vi "Do on Error.vi"(8 "error in (no error)":errorcluster, 11 "Debug UI in":refnum<class "Debug UI.lvclass">) -> ()   [LabVIEW 2018, in "Assert API Components.lvlib" / "Log Assert Core.lvlib" / "Debug UI.lvclass"]
doc: "Dynamic dispatch vi to be overriden by file or debug UI - takes the action to pass the error and handle it as required."
uses:
  Debug UI.lvclass
  C:/Program Files (x86)/National Instruments/LabVIEW 2018/vi.lib/ActorFramework/Actor/Actor.lvclass
  <vilib>/ActorFramework/Message Enqueuer/Message Enqueuer.lvclass
  Debug UI Messages/Error Data Msg/Error Data Msg.lvclass/Error Data Msg.ctl
  <vilib>/ActorFramework/Message Enqueuer/Message Enqueuer.lvclass/Message Enqueuer.ctl
  <vilib>/ActorFramework/Message Enqueuer/Enqueue.vi
  Debug UI Messages/Error Data Msg/Error Data Msg.lvclass
  C:/Program Files (x86)/National Instruments/LabVIEW 2018/vi.lib/ActorFramework/Message/Message.lvclass
  <vilib>/Utility/LVClass/Get LV Class Name.vi
  <resource>/AFDebug/Generate Trace for Message.vi
  <vilib>/ActorFramework/Message Priority Queue/Priority Enqueue.vi
  <vilib>/ActorFramework/Actor/Actor.lvclass
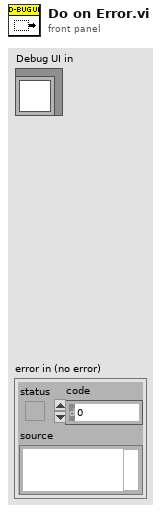
[diagram p1: front panel]
types:
  T1 = enum16{"open", "replace", "create", "open or create", "replace or create", "replace or create with confirmation"}
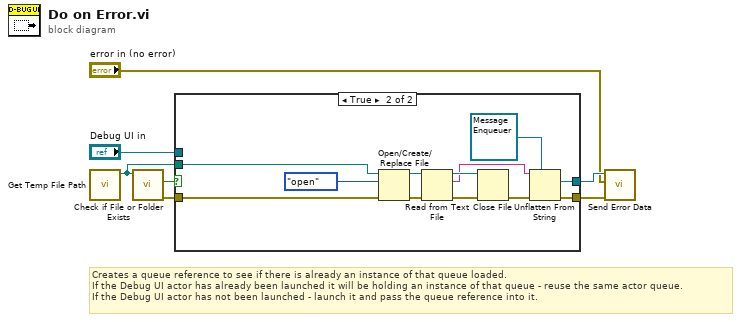
[diagram p0: block diagram]
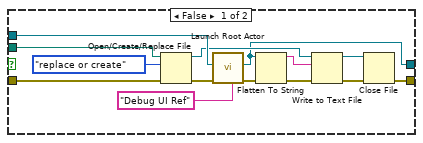
[diagram p2: hidden frame]
diagram:
  # "Creates a queue reference to see if there is already an instance of that queue loaded.\nIf the Debug UI actor has already been launched it will be holding an instance of that queue - reuse the same actor queue.\nIf the Debug UI actor has not been launched - launch it and pass the queue reference into it."
  n1 = call "Get Temp File Path.vi"() -> ("Temp File Path"=w2:path)  [unwired: 11 in]
  n2 = call <vilib>:"Check if File or Folder Exists.vi"("path"=w2) -> ("error out"=w1:errorcluster, "file or folder exists?"=w3:bool)  [unwired: 8 in, 1 out]
  n3 = case shown="True" w3 {
    tunnel: "Debug UI in" -> [w21 _]
    tunnel: [w11 w26] -> w6
    tunnel: [w15 w25] -> w4
    tunnel: w2 -> [w19 w23]
    tunnel: w1 -> [w17 w29]
    frame False {
      n4 = Open/Create/Replace File(file path (use dialog)=w19, error in=w17, operation (0:open)=T1."replace or create") -> (refnum out=w14:refnum<file>, error out=w13:errorcluster)  [unwired: 3 in, 1 out]
      n5 = call <vilib>:"Launch Root Actor.vi"("Debug Alias"="Debug UI Ref", "error in (no error)"=w13, "Actor"=w21) -> ("error out"=w10:errorcluster, "Actor's Enqueuer"=w11:refnum<class "Message Enqueuer.lvclass">)  [unwired: 7 in]
      n6 = Flatten To String(anything=w11, error in (no error)=w10) -> (data string=w8:string, error out=w9:errorcluster)  [unwired: 2 in, 1 out]
      n7 = Write to Text File(file (use dialog)=w14, text=w8, error in=w9) -> (refnum out=w12:refnum<file>, error out=w16:errorcluster)  [unwired: 1 in, 1 out]
      n8 = Close File(refnum=w12, error in=w16) -> (error out=w15:errorcluster)  [unwired: 1 out]
    }
    frame True {
      n9 = Open/Create/Replace File(file path (use dialog)=w23, error in=w29, operation (0:open)=T1."open") -> (refnum out=w33:refnum<file>, error out=w32:errorcluster)  [unwired: 3 in, 1 out]
      n10 = Read from Text File(file (use dialog)=w33, error in=w32) -> (refnum out=w31:refnum<file>, text=w28:string, error out=w30:errorcluster)  [unwired: 2 in, 1 out]
      n11 = Close File(refnum=w31, error in=w30) -> (error out=w24:errorcluster)  [unwired: 1 out]
      n12 = Unflatten From String(type=refnum<class "Message Enqueuer.lvclass"> refnum ("Actor's Enqueuer"), binary string=w28, error in (no error)=w24) -> (value=w26:refnum<class "Message Enqueuer.lvclass">, error out=w25:errorcluster)  [unwired: 2 in, 1 out]
    }
  }
  n13 = call "Send Error Data.vi"("error in (no error)"=w4, "error input"="error in (no error)", "Message Enqueuer"=w6) -> ()  [unwired: 7 in, 2 out]
